vi "sub_Extract_Packet_Boundaries - G.vi"(5 "Thresholded Signal":bool[](array[boolean])) -> (0 "packet_start_loc":i32[](array[numeric]), 3 "packet_end_loc":i32[](array[numeric]), 4 "Packet Detection Error?":bool)   [LabVIEW 2013]
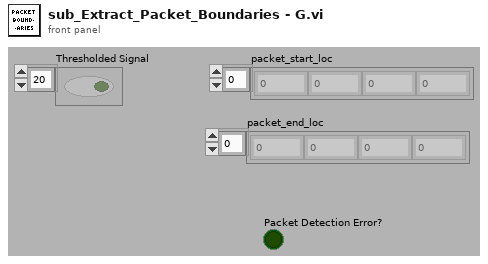
[diagram p1: front panel]
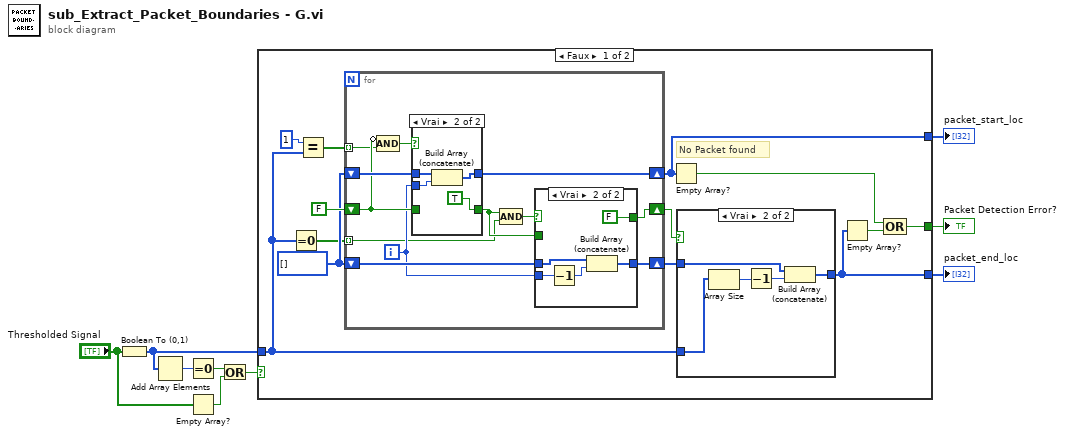
[diagram p0: block diagram]
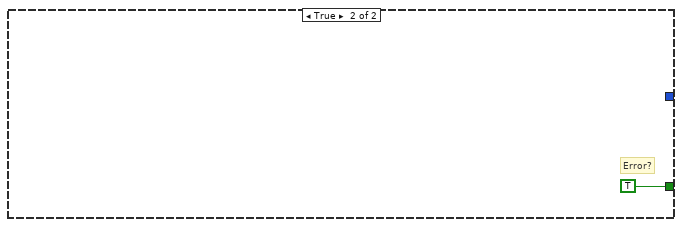
[diagram p5: hidden frame]
diagram:
  n1 = Boolean To (0,1)(Boolean="Thresholded Signal") -> (0, 1=w5:i16[])
  n2 = Add Array Elements(numeric array=w5) -> (sum=w4:i16)
  n3 = Equal To 0?(x=w4) -> (x = 0?=w2:bool)
  n4 = Empty Array?(array="Thresholded Signal") -> (empty?=w3:bool)
  n5 = Or(x=w2, y=w3) -> (x .or. y?=w1:bool)
  n6 = case shown="Faux" w1 {
    tunnel: w5 -> [w11 _]
    tunnel: [w21 TRUE] -> w7
    tunnel: [w14 _] -> w8
    tunnel: [w15 _] -> w9
    frame False {
      w18 = i32[] []
      # "No Packet found"
      n7 = Equal To 0?(x=w11) -> (x = 0?=w10:bool[])
      n8 = Equal?(x=i16 1, y=w11) -> (x = y?=w12:bool[])
      n9 = for {
        tunnel: w10 -> [w29] mode=indexing
        shift-right: [w32] -> w17
        shift-left: FALSE -> [w34]
        shift-right: [w38] -> w14
        shift-left: w18 -> [w39]
        shift-right: [w35] -> w16
        shift-left: w18 -> [w36]
        tunnel: w12 -> [w30] mode=indexing
        i -> [w31]
        n10 = Compound Arithmetic op=AND(invert w34, w30) -> (w40:bool)
        n11 = case shown="Vrai" w40 {
          tunnel: w39 -> [w49 w53]
          tunnel: [w49 w52] -> w38
          tunnel: [w48 TRUE] -> w33
          tunnel: w31 -> [_ w50]
          tunnel: w34 -> [w48 _]
          frame False {
          }
          frame True {
            n12 = Build Array (concatenate)(w53, w50) -> (w52:i32[])
          }
        }
        n13 = Compound Arithmetic op=AND(w33, w29) -> (w37:bool)
        n14 = case shown="Vrai" w37 {
          tunnel: w36 -> [w42 w47]
          tunnel: [w42 w46] -> w35
          tunnel: [w41 FALSE] -> w32
          tunnel: w31 -> [_ w44]
          tunnel: w33 -> [w41 _]
          frame False {
          }
          frame True {
            n15 = Decrement(x=w44) -> (x-1=w43:i32)
            n16 = Build Array (concatenate)(w47, w43) -> (w46:i32[])
          }
        }
      }
      n17 = Empty Array?(array=w14) -> (empty?=w22:bool)
      n18 = case shown="Vrai" w17 {
        tunnel: w16 -> [w23 w28]
        tunnel: [w23 w26] -> w15
        tunnel: w11 -> [_ w24]
        frame False {
        }
        frame True {
          n19 = Array Size(array=w24) -> (size(s)=w25:i32)
          n20 = Decrement(x=w25) -> (x-1=w27:i32)
          n21 = Build Array (concatenate)(w28, w27) -> (w26:i32[])
        }
      }
      n22 = Empty Array?(array=w15) -> (empty?=w20:bool)
      n23 = Compound Arithmetic op=OR(w22, w20) -> (w21:bool)
    }
    frame True {
      # "Error?"
    }
  }
  "Packet Detection Error?" <- w7
  "packet_end_loc" <- w9
  "packet_start_loc" <- w8
